vi "Find If Terminal Clicked Is Typedef.vi"(6 "error in (no error)":errorcluster, 9 "Terminal In":refnum<vi>) -> (0 "error out":errorcluster, 2 "Is Typedef?":T1(ring), 3 "Terminal Out":refnum<vi>, 4 "Type Definition/Class Path":string, 5 "Is Typedef/Class?":bool)   [LabVIEW 2022 SP3]
uses:
  <vilib>/Utility/Data Type/NI_Data Type.lvlib
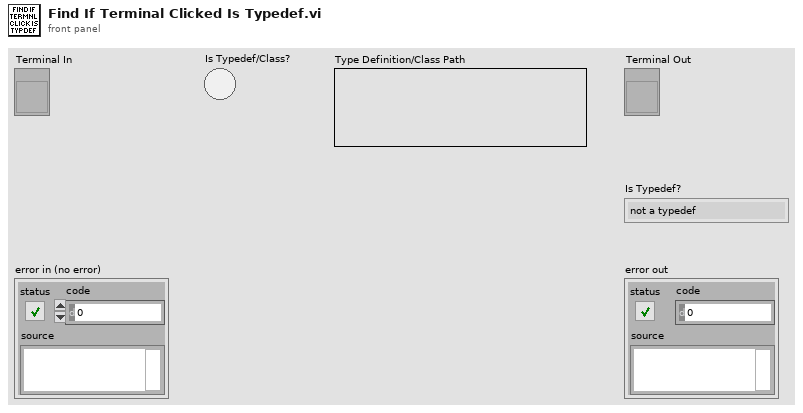
[diagram p1: front panel]
types:
  T1 = enum32{"not a typedef", "typedef", "strict typedef", "class private data"}
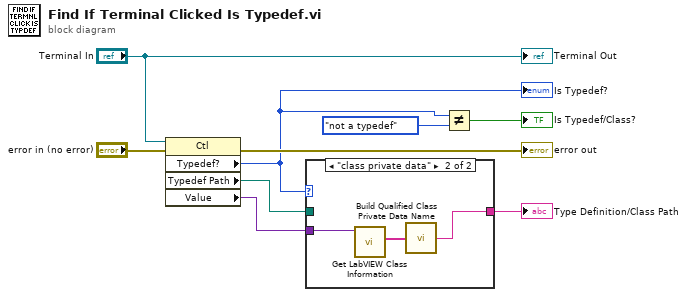
[diagram p0: block diagram]
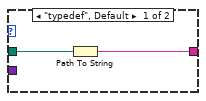
[diagram p2: hidden frame]
diagram:
  n1 = property class="Ctl"(reference="Terminal In", error in="error in (no error)") -> (error out=→"error out":errorcluster, "Typedef?"=w3:T1, "Typedef Path"=w4:path, "Value"=w1:variant)  [unwired: 1 out]
  "Is Typedef?" <- w3
  n2 = case shown="\"class private data\"" w3 {
    tunnel: w4 -> [w11 _]
    tunnel: [w10 w12] -> w2
    tunnel: w1 -> [_ w13]
    frame "typedef", Default {
      n3 = Path To String(path=w11) -> (string=w10:string)
    }
    frame "class private data" {
      n4 = call <vilib>:"Get LabVIEW Class Information.vi"("variant"=w13) -> ("qualified LabVIEW class name"=w14:string[])  [unwired: 8 in, 2 out]
      n5 = call "Build Qualified Class Private Data Name.vi"("Qualified LabVIEW Class Name"=w14) -> ("Qualified LabVIEW Class Private Data Name"=w12:string)
    }
  }
  "Type Definition/Class Path" <- w2
  n6 = Not Equal?(x=w3, y=T1."not a typedef") -> (x != y?=→"Is Typedef/Class?":bool)
  "Terminal Out" <- "Terminal In"
